vi "Do Transition.vi"(6 "Actions In":refnum<class "Iteration Actions.lvclass">, 11 "Transition in":refnum<class "Transition.lvclass">) -> (3 "Transition out":refnum<class "Transition.lvclass">, 4 "Actions":refnum<class "Iteration Actions.lvclass">)   [LabVIEW 2020, in "VolatusSeq.lvlib" / "Transition.lvclass"]
uses:
  Transition.lvclass
  Iteration Actions/Iteration Actions.lvclass
  Transition.lvclass/Transition.ctl
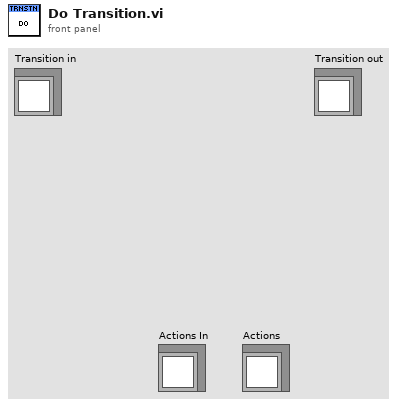
[diagram p1: front panel]
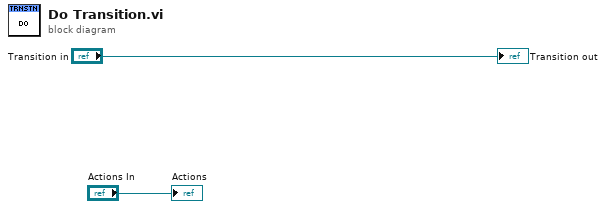
[diagram p0: block diagram]
diagram:
  "Transition out" <- "Transition in"
  "Actions" <- "Actions In"
